vi "Ke2000 Setup.vi"(6 "Set CURR Range?":u16(ring) items=["10mA", "100mA", "3A"], 8 "error in (no error)":errorcluster, 9 "Set Filter ON/OFF":bool, 10 "AUTO ON/OFF":bool, 11 "VISA resource name":refnum<visa-resource-name>) -> (0 "error out":errorcluster, 3 "VISA resource name out":refnum<visa-resource-name>)   [LabVIEW 2012]
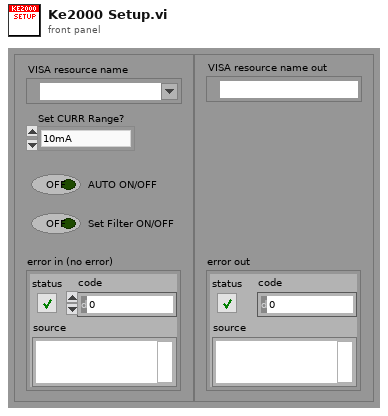
[diagram p1: front panel]
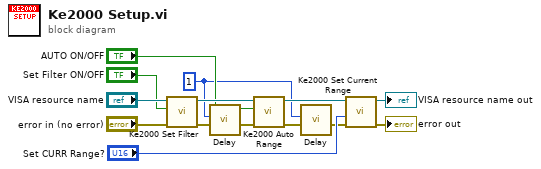
[diagram p0: block diagram]
diagram:
  w1 = u32 1 ("milliseconds to wait")
  n1 = call "Ke2000 Set Filter.vi"("error in (no error)"="error in (no error)", "Set Filter ON/OFF"="Set Filter ON/OFF", "VISA resource name"="VISA resource name") -> ("error out"=w5:errorcluster, "VISA resource name out"=w14:refnum<visa-resource-name>)  [unwired: 7 in]
  n2 = call "Delay.vi"("error in (no error)"=w5, "milliseconds to wait"=w1) -> ("error out"=w4:errorcluster)  [unwired: 9 in]
  n3 = call "Ke2000 Auto Range.vi"("error in (no error)"=w4, "AUTO ON/OFF"="AUTO ON/OFF", "VISA resource name"=w14) -> ("error out"=w3:errorcluster, "VISA resource name out"=w13:refnum<visa-resource-name>)  [unwired: 7 in]
  n4 = call "Delay.vi"("error in (no error)"=w3, "milliseconds to wait"=w1) -> ("error out"=w2:errorcluster)  [unwired: 9 in]
  n5 = call "Ke2000 Set Current Range.vi"("error in (no error)"=w2, "Set CURR Range?"="Set CURR Range?", "VISA resource name"=w13) -> ("error out"=→"error out":errorcluster, "VISA resource name out"=→"VISA resource name out":refnum<visa-resource-name>)  [unwired: 7 in]
